vi "Write AO Array.vi"(8 "error in (no error)":errorcluster, 10 "AO":T1, 11 "FPGA in":refnum<class "FPGA.lvclass">) -> (0 "error out":errorcluster, 3 "FPGA out":refnum<class "FPGA.lvclass">)   [LabVIEW 2019, in "FPGA.lvclass"]
uses:
  FPGA.lvclass
  Types/RT AOs.ctl
  FPGA.lvclass/FPGA.ctl
  <vilib>/Utility/error.llb/Error Cluster From Error Code.vi
  <vilib>/rvi/errors/niLvFpgaAdjustHostInterfaceError.vi
  <vilib>/rvi/interface/nirviReadWriteControl/nirviReadWriteControl.xnode
  FPGA VI Reference.ctl
  NiFpgaLv.dll
  <vilib>/rvi/interface/Simulation/niFpgaSimulationCallBeginRW.vi
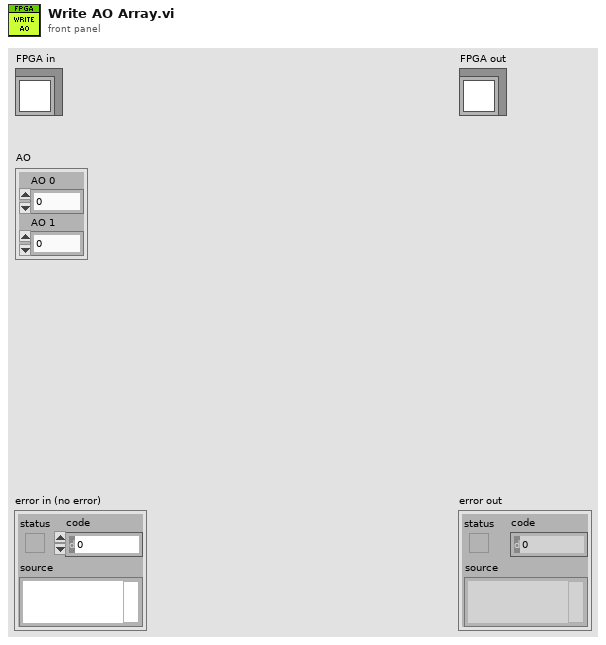
[diagram p1: front panel]
types:
  T1 = typedef "RT AOs.ctl" = cluster{"AO 0":dbl, "AO 1":dbl}
  T2 = typedef "FPGA.lvclass/FPGA VI Reference.ctl" = refnum<k20>
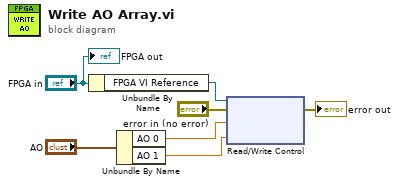
[diagram p0: block diagram]
diagram:
  n1 = Unbundle By Name("FPGA in") -> ("FPGA VI Reference"=w7:T2)
  n2 = Unbundle By Name("AO") -> ("AO 0"=w2:dbl, "AO 1"=w1:dbl)
  n3 = xnode "Read/Write Control"("FPGA VI Reference In"=w7, "error in"="error in (no error)", "Mod5/AO0"=w2, "Mod5/AO1"=w1) -> ("error out"=→"error out":errorcluster)  [unwired: 1 out]
  "FPGA out" <- "FPGA in"
